vi "FT10_Config Remove Comment.vi"(8 "error in":errorcluster, 9 "Value In":string, 10 "found? in":bool, 11 "refnum in":T1) -> (0 "error out":errorcluster, 1 "Value without Comment":string, 2 "found? out":bool, 3 "refnum out":T1)   [LabVIEW 2015]
doc: "Removes whitespace and everything after \"#\" sign which marks comments"
uses:
  <vilib>/Utility/config.llb/Config Data RefNum.ctl
  <vilib>/Utility/config.llb/NI_LVConfig.lvlib
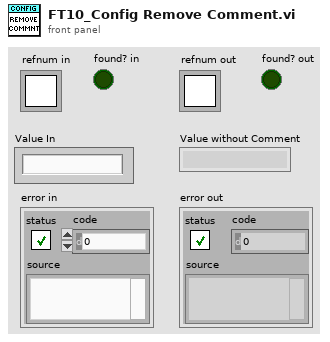
[diagram p1: front panel]
types:
  T1 = typedef "NI_LVConfig.lvlib/Config Data RefNum.ctl" = refnum<k1>
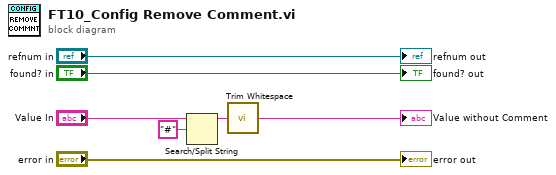
[diagram p0: block diagram]
diagram:
  n1 = Search/Split String(string="Value In", search string/char (-)="#") -> (substring before match=w5:string)  [unwired: 1 in, 2 out]
  n2 = call <vilib>:"Trim Whitespace.vi"("string"=w5) -> ("trimmed string"=→"Value without Comment":string)  [unwired: 1 in]
  "refnum out" <- "refnum in"
  "found? out" <- "found? in"
  "error out" <- "error in"
